vi "Collect and Display Data.vi"(4 "saved data comments":string, 5 "saver's name":string, 6 "saved data title":string, 7 "file name (read description)":path, 8 "error in (no error)":errorcluster, 9 "save to file":bool, 10 "data type (6 : formatted data)":u16(ring)=6 items=["raw data array 1", "raw data array 2", "raw data array 3", "raw data array 4", "error-corrected data", "error-corrected trace memory", "formatted data", "formatted memory", "formatted data / memory", "formatted data - memory"], 11 "VISA resource name":refnum<visa-resource-name>) -> (0 "error out":errorcluster, 1 "data values":cluster{"real / stim":dbl, "imag / resp":sgl}[](array[cluster]) {"imag / resp" format="%.4e"; "real / stim" format="%.4e"}, 2 "graphical display":cluster{dbl, dbl}[](graph), 3 "VISA resource name out":refnum<visa-resource-name>)   [LabVIEW 2018, in "Agilent 87XX Series.lvlib"]
doc: "It is recommended that you hold off triggers before running this VI as the HP8753 tends to \"hang\" if data is read while measurements are being taken.\n\n This VI is used to collect and display data generated by the HP8753 Network Analyzer. The VI can display error-corrected data, error-corrected trace memory, fully formatted data and memory traces. For further information on these types of data see Processsing Chain figure in the HPIB programming note. When the data type is a formatted data, the instruments screen will change to reflect what is being displayed, eg. selecting \"formatted memory\" changes the display to \"MEMORY\".\n\n The data values shown depend upon the data type and the measurement format. If the data type is \"error-corrected data\" or \"error-corrected trace memory\" and/or the measurement format is \"Smith chart\" or \"polar\", the data values are real,imaginary pairs. Otherwise the data values are stimulus,response pairs. These pairs correspond to what is shown in the graphical display.\n\n Data can also be saved to a file with this VI. When saving a file, the stimulus is always shown. The real,imaginary components or the response value are also shown depending upon the data type and the measurement format. \n\n No units are shown on the VI front panel or in the data file. All units are basic units of Hz, dB, seconds, ohms, etc. The \"saved data comments\" control should be used for any special information such as the measurement format, averaging and smoothing information, etc.\n\n Whether or not data is saved and whether the output is in real,imaginary pairs or stimulus,response parirs affects the speed of this VI. When data is saved to a file and/or when data is in stimulus,response pairs, requires the reading of the stimulus values which slows the VI down. The fastest reads are done when the data type is \"error-corrected data\" or \"error-corrected trace memory\" and/or the measurement format is \"Smith chart\" or \"polar\" and data is not being saved to a file.\n\n This VI sets the format, ie. linear or logarithmic, depending upon the sweep type. \n\nFYI - Originally this VI was written without considering the stimulus values. In most case this would be fine for display purposes as the point number could be used for the X value as most sweeps are evenly spaced. This is not the case with frequency list sweeps which can have big gaps in the sweep. For this reason the stimulus value is read (at least in the cases explained above) to make the LabVIEW display match what is display on the instrument's display."
uses:
  Agilent 87XX Series.lvlib
panel:
  # "It is recommended that you hold off triggers before running this VI as the HP8753 tends to \"hang\"\nif data is read while measurements are being taken."
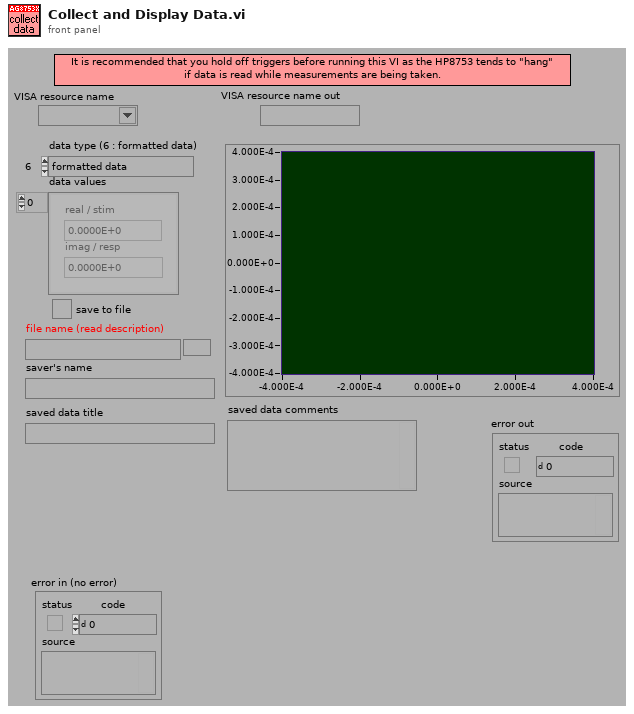
[diagram p1: front panel]
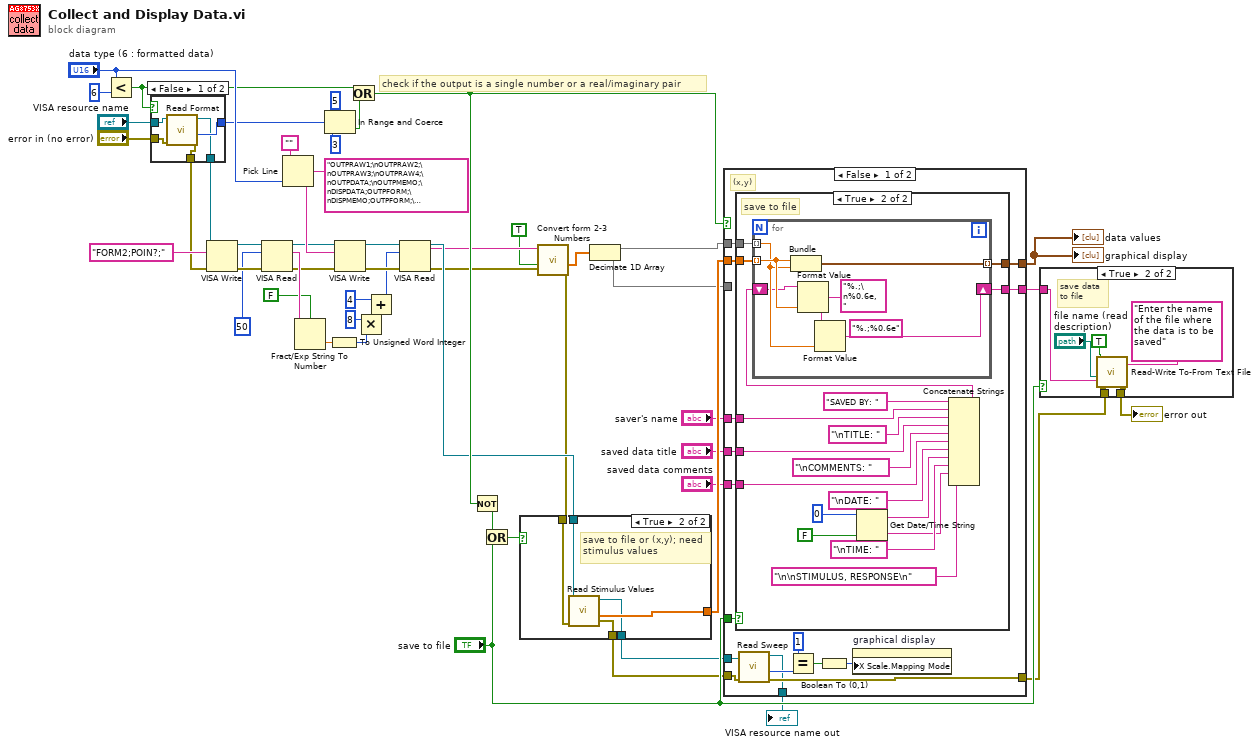
[diagram p0: block diagram]
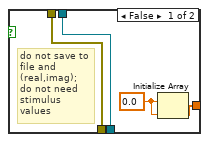
[diagram p2: hidden frame]
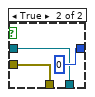
[diagram p3: hidden frame]
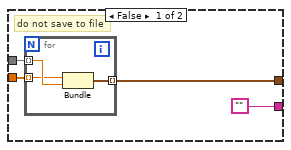
[diagram p5: hidden frame]
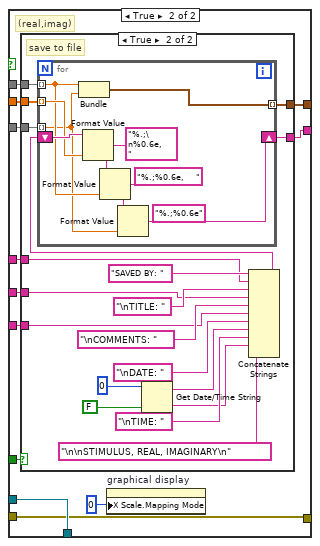
[diagram p6: hidden frame]
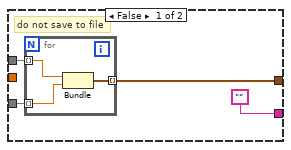
[diagram p7: hidden frame]
diagram:
  # "check if the output is a single number or a real/imaginary pair"
  n1 = Less?(x="data type (6 : formatted data)", y=u16 6) -> (x < y?=w35:bool)
  n2 = case shown="False" w35 {
    tunnel: [w58 0] -> w34
    tunnel: "VISA resource name" -> [w54 w59]
    tunnel: "error in (no error)" -> [w57 w60]
    tunnel: [w56 w59] -> w24
    tunnel: [w55 w60] -> w23
    frame False {
      n3 = call "Read Format.vi"("error in (no error)"=w57, "VISA resource name"=w54) -> ("error out"=w55:errorcluster, "format"=w58:i32, "VISA resource name out"=w56:refnum<visa-resource-name>)  [unwired: 7 in]
    }
    frame True {
    }
  }
  n4 = VISA Write(VISA resource name=w24, write buffer="FORM2;POIN?;", error in (no error)=w23) -> (VISA resource name out=w5:refnum<visa-resource-name>, error out=w50:errorcluster)  [unwired: 1 out]
  n5 = VISA Read(VISA resource name=w5, byte count=u32 50, error in (no error)=w50) -> (VISA resource name out=w32:refnum<visa-resource-name>, read buffer=w48:string, error out=w47:errorcluster)  [unwired: 1 out]
  n6 = Pick Line(string ("")="", multi-line string="OUTPRAW1;\nOUTPRAW2;\nOUTPRAW3;\nOUTPRAW4;\nOUTPDATA;\nOUTPMEMO;\nDISPDATA;OUTPFORM;\nDISPMEMO;OUTPFORM;\nDISPDDM;OUTPFORM;\nDISPDMM;OUTPFORM;", line index="data type (6 : formatted data)") -> (output string=w37:string)
  n7 = Fract/Exp String To Number(use system decimal point (T)=FALSE, string=w48) -> (number=w49:dbl)  [unwired: 2 in, 1 out]
  n8 = In Range and Coerce(upper limit=5, x=w34, lower limit=3) -> (In Range?=w51:bool)  [unwired: 1 out]
  n9 = To Unsigned Word Integer(number=w49) -> (unsigned 16bit integer=w14:u16)
  n10 = VISA Write(VISA resource name=w32, write buffer=w37, error in (no error)=w47) -> (VISA resource name out=w4:refnum<visa-resource-name>, error out=w46:errorcluster)  [unwired: 1 out]
  n11 = Or(x=w35, y=w51) -> (x .or. y?=w28:bool)
  n12 = Multiply(x=u16 8, y=w14) -> (x*y=w44:u16)
  n13 = Add(x=u16 4, y=w44) -> (x+y=w6:u16)
  n14 = VISA Read(VISA resource name=w4, byte count=w6, error in (no error)=w46) -> (VISA resource name out=w22:refnum<visa-resource-name>, read buffer=w9:string, error out=w10:errorcluster)  [unwired: 1 out]
  n15 = Not(x=w28) -> (.not. x?=w29:bool)
  n16 = Or(x=w29, y="save to file") -> (x .or. y?=w31:bool)
  n17 = call "Convert form 2-3 Numbers.vi"("error in (no error)"=w10, "data format"=TRUE, "input string"=w9) -> ("error out"=w11:errorcluster, "converted numbers"=w1:dbl[])  [unwired: 7 in]
  n18 = case shown="True" w31 {
    tunnel: w11 -> [w63 w69]
    tunnel: w22 -> [w62 w68]
    tunnel: [w65 w70] -> w27
    tunnel: [w63 w67] -> w16
    tunnel: [w62 w66] -> w17
    frame False {
      w64 = 0.0
      # "do not save to file and (real,imag);\ndo not need stimulus values"
      n19 = Initialize Array(w64, w64) -> (w65:dbl[])
    }
    frame True {
      # "save to file or (x,y); need\nstimulus values"
      n20 = call "Read Stimulus Values.vi"("error in (no error)"=w69, "VISA resource name"=w68) -> ("error out"=w67:errorcluster, "stimulus list"=w70:dbl[], "VISA resource name out"=w66:refnum<visa-resource-name>)  [unwired: 7 in]
    }
  }
  n21 = Decimate 1D Array(w1) -> (w13:dbl[], w12:dbl[])
  n22 = case shown="False" w28 {
    tunnel: w12 -> [_ w127]
    tunnel: w13 -> [w85 w130]
    tunnel: w27 -> [w84 w129]
    tunnel: [w83 w128] -> w33
    tunnel: "save to file" -> [w86 w131]
    tunnel: [w82 w126] -> w42
    tunnel: "saver's name" -> [w81 w125]
    tunnel: "saved data title" -> [w80 w124]
    tunnel: "saved data comments" -> [w79 w123]
    tunnel: w16 -> [w78 w121]
    tunnel: w17 -> [w77 w122]
    tunnel: [w72 w121] -> w15
    tunnel: [w71 w122] -> w3
    frame False {
      # "(x,y)"
      n23 = case shown="True" w86 {
        tunnel: w85 -> [w90 w111]
        tunnel: w84 -> [w89 w110]
        tunnel: [w88 w99] -> w83
        tunnel: ["" w98] -> w82
        tunnel: w81 -> [_ w97]
        tunnel: w80 -> [_ w96]
        tunnel: w79 -> [_ w95]
        frame False {
          # "do not save to file"
          n24 = for {
            tunnel: w90 -> [w92] mode=indexing
            tunnel: [w93] -> w88 mode=indexing
            tunnel: w89 -> [w91] mode=indexing
            n25 = Bundle(w91, w92) -> (w93:cluster{dbl, dbl})  [unwired: 1 in]
          }
        }
        frame True {
          # "save to file"
          n26 = Get Date/Time String(date format (0)=0, want seconds? (F)=FALSE) -> (date string=w103:string, time string=w101:string)  [unwired: 1 in]
          n27 = Concatenate Strings("SAVED BY: ", w97, "\nTITLE: ", w96, "\nCOMMENTS: ", w95, "\nDATE: ", w103, "\nTIME: ", w101, "\n\nSTIMULUS, RESPONSE\n") -> (w100:string)
          n28 = for {
            tunnel: w111 -> [w114] mode=indexing
            tunnel: [w119] -> w99 mode=indexing
            tunnel: w110 -> [w115] mode=indexing
            shift-right: [w112] -> w98
            shift-left: w100 -> [w113]
            n29 = Bundle(w115, w114) -> (w119:cluster{dbl, dbl})  [unwired: 1 in]
            n30 = Format Value(string ("")=w113, format string="%.;\n%0.6e,  ", value (0)=w115) -> (output string=w116:string)
            n31 = Format Value(string ("")=w116, format string="%.;%0.6e", value (0)=w114) -> (output string=w112:string)
          }
        }
      }
      n32 = call "Read Sweep.vi"("error in (no error)"=w78, "VISA resource name"=w77) -> ("error out"=w72:errorcluster, "sweep type"=w76:i32, "VISA resource name out"=w71:refnum<visa-resource-name>)  [unwired: 7 in]
      n33 = Equal?(x=1, y=w76) -> (x = y?=w74:bool)
      n34 = Boolean To (0,1)(Boolean=w74) -> (0, 1=w73:i16)
      n35 = property on="graphical display" class="XYGraph (strict)"("X Scale.Mapping Mode"=w73) -> ()  [unwired: 2 in, 2 out]
    }
    frame True {
      # "(real,imag)"
      n36 = case shown="True" w131 {
        tunnel: w130 -> [w135 w157]
        tunnel: w129 -> [_ w144]
        tunnel: [w134 w143] -> w128
        tunnel: ["" w146] -> w126
        tunnel: w127 -> [w132 w145]
        tunnel: w125 -> [_ w142]
        tunnel: w124 -> [_ w141]
        tunnel: w123 -> [_ w140]
        frame False {
          # "do not save to file"
          n37 = for {
            tunnel: w135 -> [w137] mode=indexing
            tunnel: [w138] -> w134 mode=indexing
            tunnel: w132 -> [w136] mode=indexing
            n38 = Bundle(w137, w136) -> (w138:cluster{dbl, dbl})  [unwired: 1 in]
          }
        }
        frame True {
          # "save to file"
          n39 = Get Date/Time String(date format (0)=0, want seconds? (F)=FALSE) -> (date string=w150:string, time string=w148:string)  [unwired: 1 in]
          n40 = Concatenate Strings("SAVED BY: ", w142, "\nTITLE: ", w141, "\nCOMMENTS: ", w140, "\nDATE: ", w150, "\nTIME: ", w148, "\n\nSTIMULUS, REAL, IMAGINARY\n") -> (w147:string)
          n41 = for {
            tunnel: w157 -> [w159] mode=indexing
            tunnel: [w168] -> w143 mode=indexing
            shift-right: [w160] -> w146
            shift-left: w147 -> [w164]
            tunnel: w145 -> [w158] mode=indexing
            tunnel: w144 -> [w163] mode=indexing
            n42 = Bundle(w159, w158) -> (w168:cluster{dbl, dbl})  [unwired: 1 in]
            n43 = Format Value(string ("")=w164, format string="%.;\n%0.6e,    ", value (0)=w163) -> (output string=w165:string)
            n44 = Format Value(string ("")=w165, format string="%.;%0.6e,    ", value (0)=w159) -> (output string=w161:string)
            n45 = Format Value(string ("")=w161, format string="%.;%0.6e", value (0)=w158) -> (output string=w160:string)
          }
        }
      }
      n46 = property on="graphical display" class="XYGraph (strict)"("X Scale.Mapping Mode"=u8 0) -> ()  [unwired: 2 in, 2 out]
    }
  }
  "data values" <- w33
  "graphical display" <- w33
  "VISA resource name out" <- w3
  n47 = case shown="True" "save to file" {
    tunnel: w42 -> [_ w172]
    tunnel: w15 -> [w169 w171]
    tunnel: [w169 w170] -> w21
    frame False {
    }
    frame True {
      # "save data to file"
      n48 = call "Read-Write To-From Text File.vi"("string to be written"=w172, "dialog box prompt"="Enter the name of the file where the data is to be saved", "error in (no error)"=w171, "file name (read description)"="file name (read description)", "read/write (f:read)"=TRUE) -> ("error out"=w170:errorcluster)  [unwired: 5 in, 1 out]
    }
  }
  "error out" <- w21
